vi "DSF.Engine.Execution.BuilderManager.New.vi"(8 "error in (no error)":errorcluster, 11 "Framework Cache":refnum<class "DSF.Engine.Memory.Cache.Framework.lvclass">) -> (0 "error out":errorcluster, 3 "Builder Manager out":refnum<class "DSF.Engine.Execution.BuilderManager.lvclass">)   [LabVIEW 2016, in "DSF.Engine.lvlib" / "DSF.Engine.Execution.BuilderManager.lvclass"]
uses:
  DSF.Engine.Execution.BuilderManager.lvclass
  Cache/DSF.Engine.Memory.Cache.Framework.lvclass
  Cache/DSF.Engine.Memory.Cache.Framework.lvclass/DSF.Engine.Memory.Cache.Framework.ctl
  Builder/DSF.Engine.Execution.Builder.lvclass/DSF.Engine.Execution.Builder.ctl
  DSF.Engine.Execution.BuilderManager.lvclass/DSF.Engine.Execution.BuilderManager.ctl
  Builder/DSF.Engine.Execution.Builder.Set FIFOs.vi
  Builder/DSF.Engine.Execution.Builder.Set Status Pointers.vi
  Submodules/Memory/Source/Classes/Standard Types/Memory.Pointer.U32.New.vi
  Builder/DSF.Engine.Execution.Builder.Set Framework Cache.vi
  Submodules/Memory/Source/Classes/Standard Types/Memory.Pointer.U32.lvclass
  C:/Git/SourceTree/DSF/Source/Submodules/Memory/Source/Classes/Internal/Memory.Pointer.Internal.lvclass
  Submodules/Memory/Source/Classes/Internal/Memory.Pointer.Internal.Allocate.vi
  Builder/DSF.Engine.Execution.Builder.lvclass
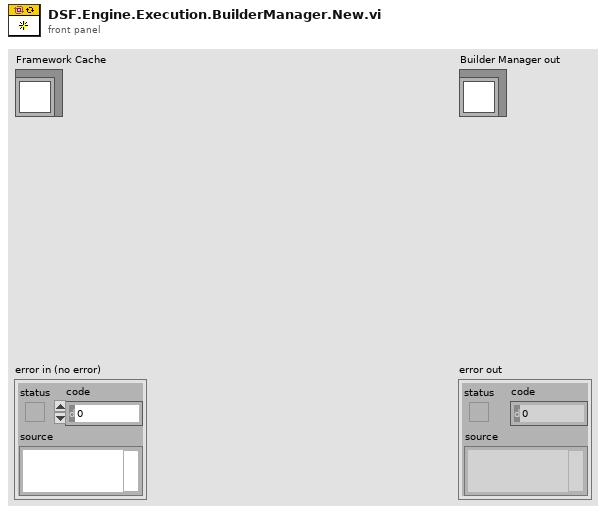
[diagram p1: front panel]
types:
  T1 = typedef "DSF.Engine.lvlib/DSF.Engine.Runtime.Framework.lvclass/DSF.Engine.Runtime.Framework.Hardware.ctl" = cluster{"CPU":T2}
  T2 = typedef "DSF.Engine.lvlib/DSF.Engine.Typedefs.CPU Info.ctl" = cluster{"core count":i32, "caches":cluster{"total cache size":i32, "cache entry size":i32}[]}
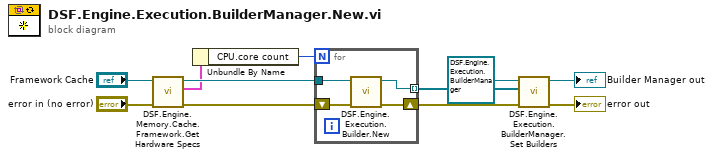
[diagram p0: block diagram]
diagram:
  n1 = call "DSF.Engine.Memory.Cache.Framework.Get Hardware Specs.vi"("error in (no error)"="error in (no error)", "Framework Cache in"="Framework Cache") -> ("error out"=w2:errorcluster, "Hardware Info"=w1:T1, "Framework Cache out"=w3:refnum<class "DSF.Engine.Memory.Cache.Framework.lvclass">)  [unwired: 7 in]
  n2 = Unbundle By Name(w1) -> ("CPU.core count"=w4:i32)
  n3 = for {
    N: w4 -> [_]
    shift-right: [w14] -> w8
    shift-left: w2 -> [w15]
    tunnel: [w13] -> w7 mode=indexing
    tunnel: w3 -> [w12]
    n4 = call "DSF.Engine.Execution.Builder.New.vi"("error in (no error)"=w15, "Framework Cache"=w12) -> ("error out"=w14:errorcluster, "Builder"=w13:refnum<class "DSF.Engine.Execution.Builder.lvclass">)  [unwired: 8 in]
  }
  n5 = call "DSF.Engine.Execution.BuilderManager.Set Builders.vi"("error in (no error)"=w8, "Builders"=w7, "Builder Manager in"=refnum<class "DSF.Engine.Execution.BuilderManager.lvclass"> refnum) -> ("error out"=→"error out":errorcluster, "Builder Manager out"=→"Builder Manager out":refnum<class "DSF.Engine.Execution.BuilderManager.lvclass">)  [unwired: 7 in]
